vi "SRTS_Save.vi"(8 "error in":errorcluster, 11 "TDMS in":refnum<class "TDMS.lvclass">) -> (0 "error out":errorcluster, 3 "TDMS out":refnum<class "TDMS.lvclass">)   [LabVIEW 2017, in "Report_lib.lvlib" / "TDMS.lvclass"]
uses:
  TDMS.lvclass
  Controller/Controls/Controller DAQ Data.ctl
  TDMS.lvclass/TDMS.ctl
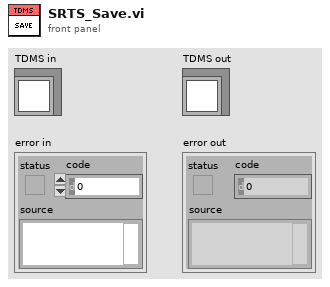
[diagram p1: front panel]
types:
  T1 = typedef "Controller DAQ Data.ctl" = cluster{"AOM data":dbl[], "AIMV data":dbl[], "AIMC data":dbl[], "DOM data":dbl[], "DIM data":dbl[], "AOM timestamp":dbl, "AIMV timestamp":dbl, "AIMC timestamp":dbl, "DOM timestamp":dbl, "DIM timestamp":dbl}
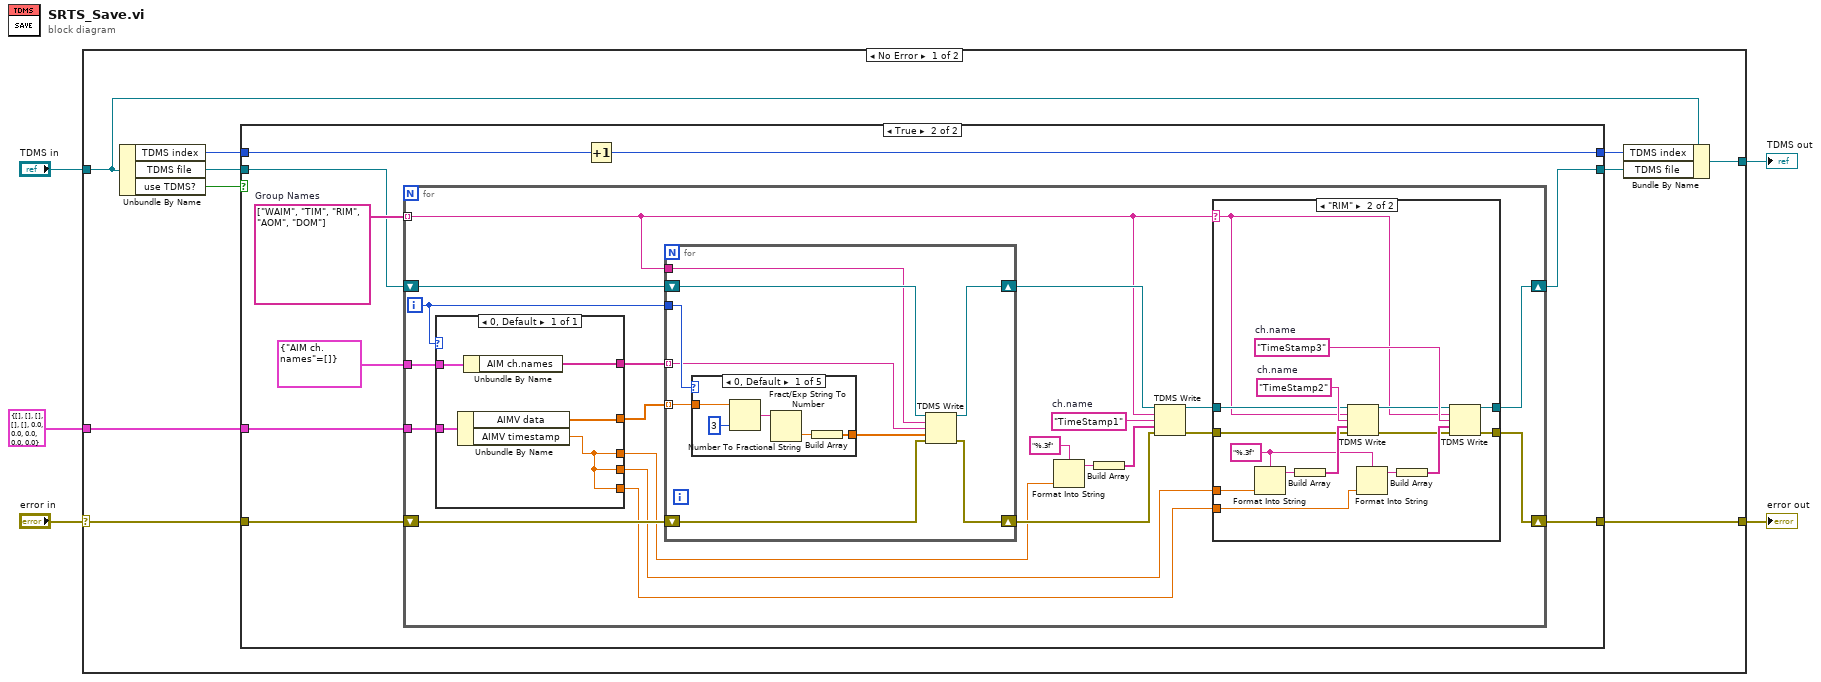
[diagram p0: block diagram]
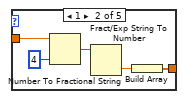
[diagram p4: hidden frame]
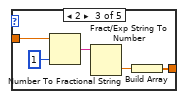
[diagram p5: hidden frame]
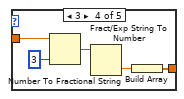
[diagram p6: hidden frame]
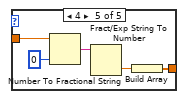
[diagram p7: hidden frame]
diagram:
  n1 = case shown="No Error" "error in" {
    selector: "error in" -> [w14 w107]
    tunnel: [w7 w107] -> w2
    tunnel: [w9 w106] -> w3
    tunnel: "TDMS in" -> [w10 w106]
    tunnel: T1 {"AOM data"=[], "AIMV data"=[], "AIMC data"=[], "DOM data"=[], "DIM data"=[], "AOM timestamp"=0.0, "AIMV timestamp"=0.0, "AIMC timestamp"=0.0, "DOM timestamp"=0.0, "DIM timestamp"=0.0} ("DAQ Data") -> [w8 _]
    frame No Error {
      n2 = Unbundle By Name(w10) -> ("TDMS index"=w13:i32, "TDMS file"=w15:refnum<k34>, "use TDMS?"=w6:bool)
      n3 = case shown="True" w6 {
        tunnel: w15 -> [w17 w26]
        tunnel: w14 -> [w16 w25]
        tunnel: w13 -> [w18 w24]
        tunnel: [w18 w23] -> w12
        tunnel: [w17 w22] -> w11
        tunnel: w8 -> [_ w21]
        tunnel: [w16 w20] -> w7
        frame False {
        }
        frame True {
          w27 = string[] ["WAIM", "TIM", "RIM", "AOM", "DOM"]  # Group Names
          n4 = for {
            tunnel: w27 -> [w34] mode=indexing
            tunnel: cluster{"AIM ch.names":string[]} {"AIM ch.names"=[]} -> [w47]
            tunnel: w21 -> [w48]
            shift-right: [w30] -> w22
            shift-left: w26 -> [w43]
            shift-right: [w31] -> w20
            shift-left: w25 -> [w42]
            i -> [w44]
            w41 = "TimeStamp1"  # ch.name
            n5 = case shown="0, Default" w44 {
              tunnel: w48 -> [w71]
              tunnel: w47 -> [w70]
              tunnel: [w69] -> w46
              tunnel: [w68] -> w45
              tunnel: [w67] -> w36
              tunnel: [w67] -> w29
              tunnel: [w67] -> w28
              frame 0, Default {
                n6 = Unbundle By Name(w71) -> ("AIMV data"=w69:dbl[], "AIMV timestamp"=w67:dbl)
                n7 = Unbundle By Name(w70) -> ("AIM ch.names"=w68:string[])
              }
            }
            n8 = for {
              tunnel: w46 -> [w79] mode=indexing
              tunnel: w45 -> [w76] mode=indexing
              tunnel: w44 -> [w80]
              shift-right: [w77] -> w38
              shift-left: w43 -> [w78]
              tunnel: w34 -> [w75]
              shift-right: [w72] -> w39
              shift-left: w42 -> [w73]
              n9 = case shown="0, Default" w80 {
                tunnel: w79 -> [w82 w87 w92 w97 w102]
                tunnel: [w81 w86 w91 w96 w101] -> w74
                frame 0, Default {
                  n10 = Number To Fractional String(number=w82, precision (6)=i16 3) -> (F-format string=w84:string)  [unwired: 2 in]
                  n11 = Fract/Exp String To Number(string=w84) -> (number=w85:dbl)  [unwired: 3 in, 1 out]
                  n12 = Build Array(w85) -> (w81:dbl[])
                }
                frame 1 {
                  n13 = Number To Fractional String(number=w87, precision (6)=i16 4) -> (F-format string=w89:string)  [unwired: 2 in]
                  n14 = Fract/Exp String To Number(string=w89) -> (number=w90:dbl)  [unwired: 3 in, 1 out]
                  n15 = Build Array(w90) -> (w86:dbl[])
                }
                frame 2 {
                  n16 = Number To Fractional String(number=w92, precision (6)=i16 1) -> (F-format string=w94:string)  [unwired: 2 in]
                  n17 = Fract/Exp String To Number(string=w94) -> (number=w95:dbl)  [unwired: 3 in, 1 out]
                  n18 = Build Array(w95) -> (w91:dbl[])
                }
                frame 3 {
                  n19 = Number To Fractional String(number=w97, precision (6)=i16 3) -> (F-format string=w99:string)  [unwired: 2 in]
                  n20 = Fract/Exp String To Number(string=w99) -> (number=w100:dbl)  [unwired: 3 in, 1 out]
                  n21 = Build Array(w100) -> (w96:dbl[])
                }
                frame 4 {
                  n22 = Number To Fractional String(number=w102, precision (6)=i16 0) -> (F-format string=w104:string)  [unwired: 2 in]
                  n23 = Fract/Exp String To Number(string=w104) -> (number=w105:dbl)  [unwired: 3 in, 1 out]
                  n24 = Build Array(w105) -> (w101:dbl[])
                }
              }
              n25 = TDMS Write(0:w78, 5:w75, 7:w76, 9:w74, 11:w73) -> (4:w77:refnum<k34>, 15:w72:errorcluster)  [unwired: 1 in, 2 out]
            }
            n26 = Format Into String(format string="%.3f", w36) -> (resulting string=w35:string)  [unwired: 2 in, 1 out]
            n27 = Build Array(w35) -> (w40:string[])
            n28 = TDMS Write(0:w38, 5:w34, 7:w41, 9:w40, 11:w39) -> (4:w33:refnum<k34>, 15:w32:errorcluster)  [unwired: 1 in, 2 out]
            n29 = case shown="\"RIM\"" w34 {
              selector: w34 -> [_ w54]
              tunnel: w33 -> [w49 w63]
              tunnel: w32 -> [w50 w62]
              tunnel: [w50 w55] -> w31
              tunnel: [w49 w56] -> w30
              tunnel: w29 -> [_ w53]
              tunnel: w28 -> [_ w52]
              frame Default {
              }
              frame "RIM" {
                w61 = "TimeStamp3"  # ch.name
                w51 = "%.3f" ("format string")
                w64 = "TimeStamp2"  # ch.name
                n30 = Format Into String(format string=w51, w53) -> (resulting string=w66:string)  [unwired: 2 in, 1 out]
                n31 = Build Array(w66) -> (w65:string[])
                n32 = TDMS Write(0:w63, 5:w54, 7:w64, 9:w65, 11:w62) -> (4:w58:refnum<k34>, 15:w57:errorcluster)  [unwired: 1 in, 2 out]
                n33 = Format Into String(format string=w51, w52) -> (resulting string=w59:string)  [unwired: 2 in, 1 out]
                n34 = Build Array(w59) -> (w60:string[])
                n35 = TDMS Write(0:w58, 5:w54, 7:w61, 9:w60, 11:w57) -> (4:w56:refnum<k34>, 15:w55:errorcluster)  [unwired: 1 in, 2 out]
              }
            }
          }
          n36 = Increment(x=w24) -> (x+1=w23:i32)
        }
      }
      n37 = Bundle By Name(cluster=w10, "TDMS index"=w12, "TDMS file"=w11) -> (w9:refnum<class "TDMS.lvclass">)
    }
    frame Error {
    }
  }
  "error out" <- w2
  "TDMS out" <- w3
